vi "LC_PV_global.vi"() -> ()   [LabVIEW 2016]
panel:
  in  "Digital control channel number":dbl
  in  "Digital statues channel number":dbl
  in  "Analogue control channel number":dbl
  in  "Analogue statues channel number":dbl
  in  "DNP3 Outstation Address":dbl
  in  "DNP3 Master Address":dbl
  in  "DNP3 port":dbl
  in  "IP_PV":dbl[](array[numeric])
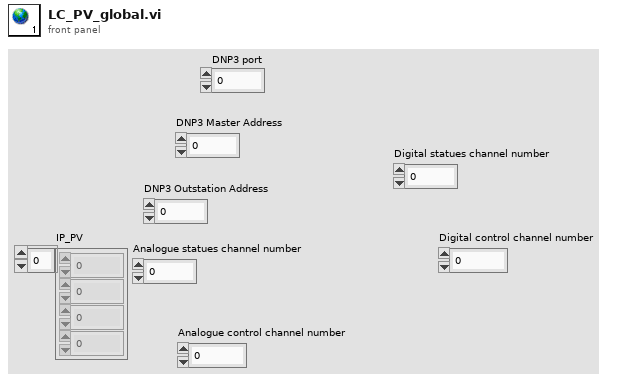
[diagram p1: front panel]
diagram:
